vi "Get-exit.vi"(8 "error in (no error)":errorcluster, 11 "UI ref. in":refnum<data-value>) -> (0 "error out":errorcluster, 1 "Exit?":bool, 3 "UI ref.":refnum<data-value>)   [LabVIEW 2013, in "CameraVision.lvlib" / "CV-UI.lvclass"]
uses:
  CV-UI.lvclass
  CV-UI.lvclass/CV-UI.ctl
  Read Exit.vi
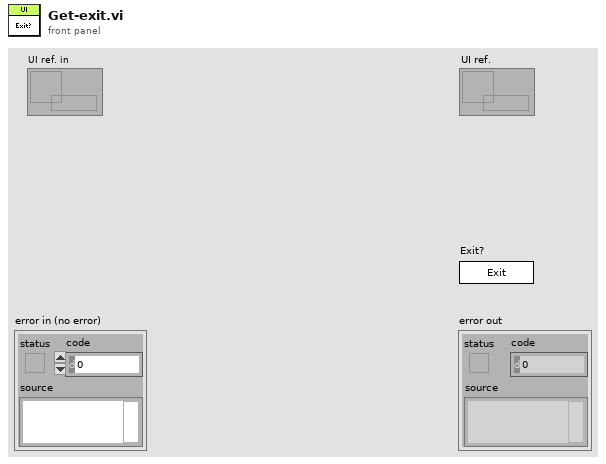
[diagram p1: front panel]
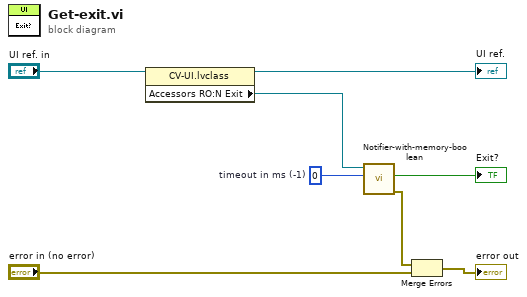
[diagram p0: block diagram]
diagram:
  w5 = 0  # timeout in ms (-1)
  n1 = property class="CV-UI.lvclass"(reference="UI ref. in") -> (reference out=→"UI ref.":refnum<data-value>, "Accessors RO:N Exit"=w4:refnum<notifier>)  [unwired: 1 in, 1 out]
  n2 = call "Notifier-with-memory-boolean.vi"("Timeout [ms]"=w5, "Notifier in"=w4) -> ("error IO"=w3:errorcluster, "Notification"=→"Exit?":bool)  [unwired: 8 in]
  n3 = Merge Errors(w3, "error in (no error)") -> (→"error out":errorcluster)
